vi "Add Language.vi"(8 "error in (no error)":errorcluster, 10 "Language":T1, 11 "LangFile in":refnum<class "Resource Data.lvclass">) -> (0 "error out":errorcluster, 3 "LangFile out":refnum<class "Resource Data.lvclass">)   [LabVIEW 2013, in "SET Project Data.lvlib" / "Resource Data.lvclass"]
uses:
  Resource Data.lvclass
  Types/ProjFile_Language Entry.ctl
  Resource Data.lvclass/Resource Data.ctl
  SET Project Data.lvlib
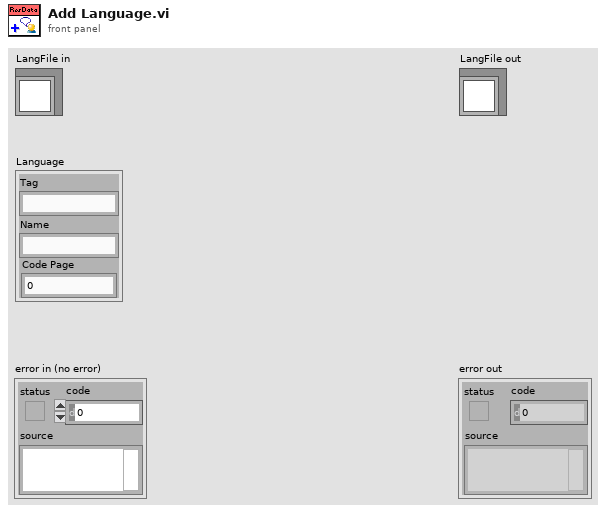
[diagram p1: front panel]
types:
  T1 = typedef "SET Project Data.lvlib/ProjFile_Language Entry.ctl" = cluster{"Tag":string, "Name":string, "Code Page":u16}
  T2 = typedef "SET Project Data.lvlib/ProjFile_Resource Entry.ctl" = cluster{"RID":string, "Tag":string, "Strings [] (UTF-16)":string[], "Shared?":bool}
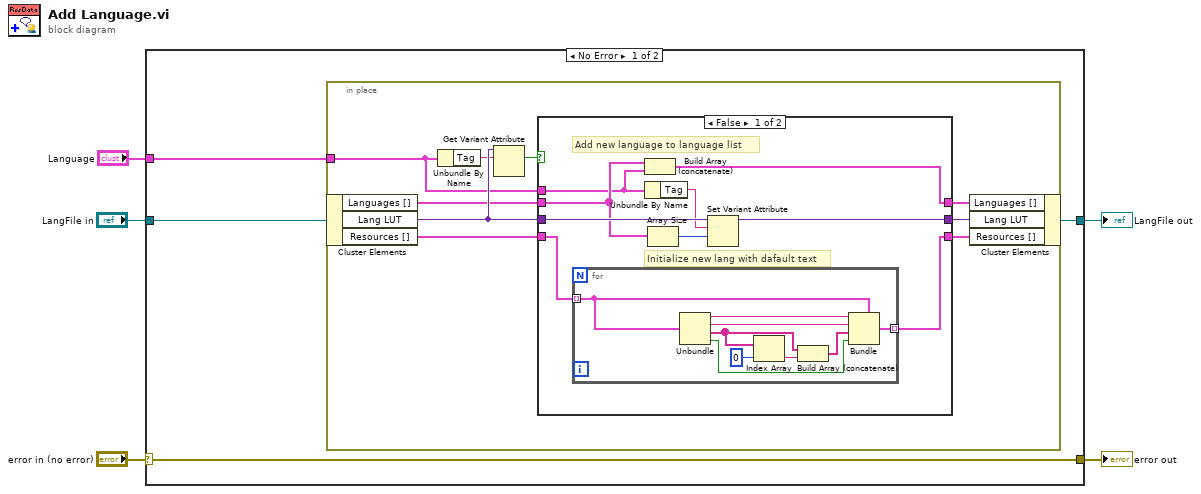
[diagram p0: block diagram]
diagram:
  n1 = case shown="No Error" "error in (no error)" {
    selector: "error in (no error)" -> [w9 w41]
    tunnel: [w9 w41] -> w4
    tunnel: [w8 w40] -> w3
    tunnel: "LangFile in" -> [w6 w40]
    tunnel: "Language" -> [w7 _]
    frame No Error {
      n2 = in-place {
        in-place-border: w7 -> [w11]
        n3 = in-place-cluster #1(w6) -> ("Languages []"=w13:T1[], "Lang LUT"=w15:variant, "Resources []"=w18:T2[])
        n4 = Unbundle By Name(w11) -> ("Tag"=w10:string)
        n5 = Get Variant Attribute(Variant=w15, name=w10) -> (found=w14:bool)  [unwired: 2 in, 3 out]
        n6 = case shown="False" w14 {
          tunnel: w18 -> [w27 w39]
          tunnel: [w26 w39] -> w17
          tunnel: [w24 w38] -> w16
          tunnel: w15 -> [w25 w38]
          tunnel: w11 -> [w20 _]
          tunnel: w13 -> [w22 w37]
          tunnel: [w23 w37] -> w12
          frame False {
            # "Add new language to language list"
            # "Initialize new lang with dafault text"
            n7 = for {
              tunnel: w27 -> [w34] mode=indexing
              tunnel: [w33] -> w26 mode=indexing
              n8 = Unbundle(w34) -> ("RID"=w36:string, "Tag"=w35:string, "Strings [] (UTF-16)"=w31:string[], "Shared?"=w28:bool)
              n9 = Index Array(array=w31, index=0) -> (element=w29:string)
              n10 = Build Array (concatenate)(w31, w29) -> (w32:string[])
              n11 = Bundle(cluster=w34, "RID"=w36, "Tag"=w35, "Strings [] (UTF-16)"=w32, "Shared?"=w28) -> (w33:T2)
            }
            n12 = Build Array (concatenate)(w22, w20) -> (w23:T1[])
            n13 = Unbundle By Name(w20) -> ("Tag"=w19:string)
            n14 = Array Size(array=w22) -> (size(s)=w21:i32)
            n15 = Set Variant Attribute(Variant=w25, name=w19, value=w21) -> (Variant out=w24:variant)  [unwired: 1 in, 2 out]
          }
          frame True {
            # "Don't allow duplicates"
          }
        }
        n16 = in-place-cluster #1("Languages []"=w12, "Lang LUT"=w16, "Resources []"=w17) -> (w8:refnum<class "Resource Data.lvclass">)
      }
    }
    frame Error {
    }
  }
  "error out" <- w4
  "LangFile out" <- w3
